vi "Msg - Send.vi"(0 "Message":T1, 7 "High Priority?":bool, 11 "error in (no error)":errorcluster) -> (15 "error out":errorcluster)   [LabVIEW 2017, in "Error Handler - Logger.lvlib"]
doc: "Send Messages to this Module."
uses:
  Error Handler - Logger.lvlib
  Controls/Message.ctl
  Controls/Module - States.ctl
  Modules.ctl
  Controls/Message - Queue Manager Mode.ctl
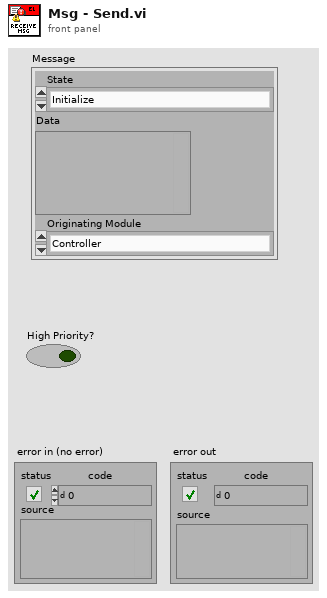
[diagram p1: front panel]
types:
  T1 = typedef "Error Handler - Logger.lvlib/Message.ctl" = cluster{"State":T2, "Data":variant, "Originating Module":T3}
  T2 = typedef "Error Handler - Logger.lvlib/Module - States.ctl" = enum16{"Initialize", "Event ", "Send data", "FP Element: Update", "FP Element: Disable/Enable", "Timer: Setup", "Terminate", "--------Template----------", "Process Error", "Log ", "Log Error"}
  T3 = typedef "Error Handler - Logger.lvlib/Modules.ctl" = enum16{"Controller", "Error Handler - Logger"}
  T4 = typedef "Error Handler - Logger.lvlib/Message - Queue Manager Mode.ctl" = enum16{"Create", "Get", "Destroy"}
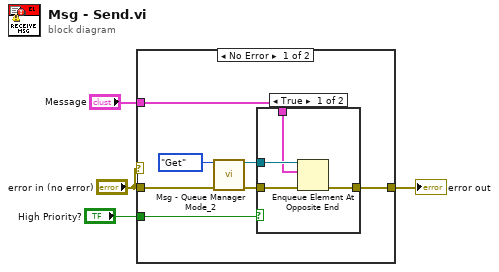
[diagram p0: block diagram]
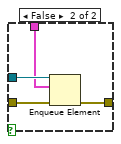
[diagram p2: hidden frame]
diagram:
  n1 = case shown="No Error" "error in (no error)" {
    tunnel: [w8 w20] -> w4
    tunnel: "error in (no error)" -> [w9 w20]
    tunnel: "Message" -> [w6 _]
    tunnel: "High Priority?" -> [w5 _]
    frame No Error {
      n2 = call "Msg - Queue Manager Mode_2.vi"("Mode"=Message_-_Queue_Manager_Mode."Get", "error in (no error)"=w9) -> (">>ThisModule"=w7:refnum<queue>, "error out"=w10:errorcluster)  [unwired: 11 in, 1 out]
      n3 = case shown="True" w5 {
        tunnel: w10 -> [w15 w19]
        tunnel: [w14 w18] -> w8
        tunnel: w7 -> [w13 w17]
        tunnel: w6 -> [w12 w16]
        frame True {
          n4 = Enqueue Element At Opposite End(queue=w13, element=w12, error in (no error)=w15) -> (error out=w14:errorcluster)  [unwired: 1 in, 2 out]
        }
        frame False {
          n5 = Enqueue Element(queue=w17, element=w16, error in (no error)=w19) -> (error out=w18:errorcluster)  [unwired: 1 in, 2 out]
        }
      }
    }
    frame Error {
    }
  }
  "error out" <- w4
